vi "Input_Sensors_Conveyor.vi"(10 "IR Upper Limit Threshold":dbl=3.0, 11 "IR Distance Threshold":dbl=5.0) -> (0 "Conveyor Sensor Inputs":T2, 3 "ConveyorV2 Inputs":T1)   [LabVIEW 2012]
uses:
  Sensor_Input_Conveyor.ctl
  Sensor_Input_ConveyorV2.ctl
panel:
  out "error out":errorcluster
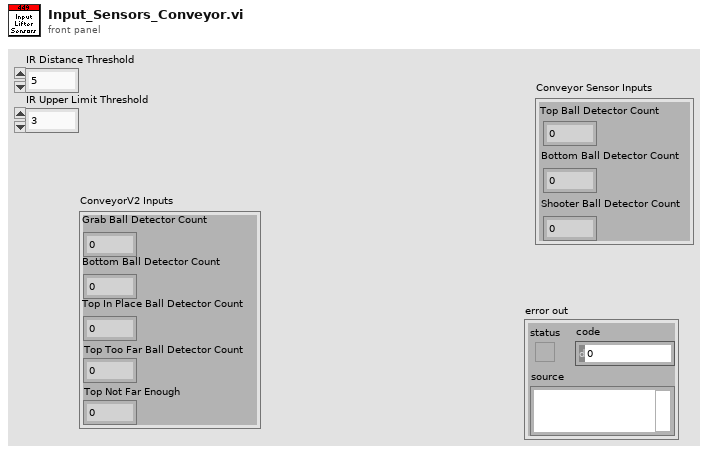
[diagram p1: front panel]
types:
  T1 = typedef "Sensor_Input_ConveyorV2.ctl" = cluster{"Grab Ball Detector Count":i32, "Bottom Ball Detector Count":i32, "Top In Place Ball Detector Count":i32, "Top Too Far Ball Detector Count":i32, "Top Not Far Enough":i32}
  T2 = typedef "Sensor_Input_Conveyor.ctl" = cluster{"Top Ball Detector Count":i32, "Bottom Ball Detector Count":i32, "Shooter Ball Detector Count":i32}
  T3 = typedef "WPI_DigitalInputDevRef.ctl" = cluster{"DevStatus":errorcluster, "DIO Channel":T4, "Digital Module":T5}
  T4 = typedef "FPGA_DIOChannel.ctl" = enum8{"DIO 1", "DIO 2", "DIO 3", "DIO 4", "DIO 5", "DIO 6", "DIO 7", "DIO 8", "DIO 9", "DIO 10", "DIO 11", "DIO 12", "DIO 13", "DIO 14", "Invalid"}
  T5 = typedef "FPGA_TypedefDigitalModule.ctl" = enum16{"Digital Module 1", "Digital Module 2"}
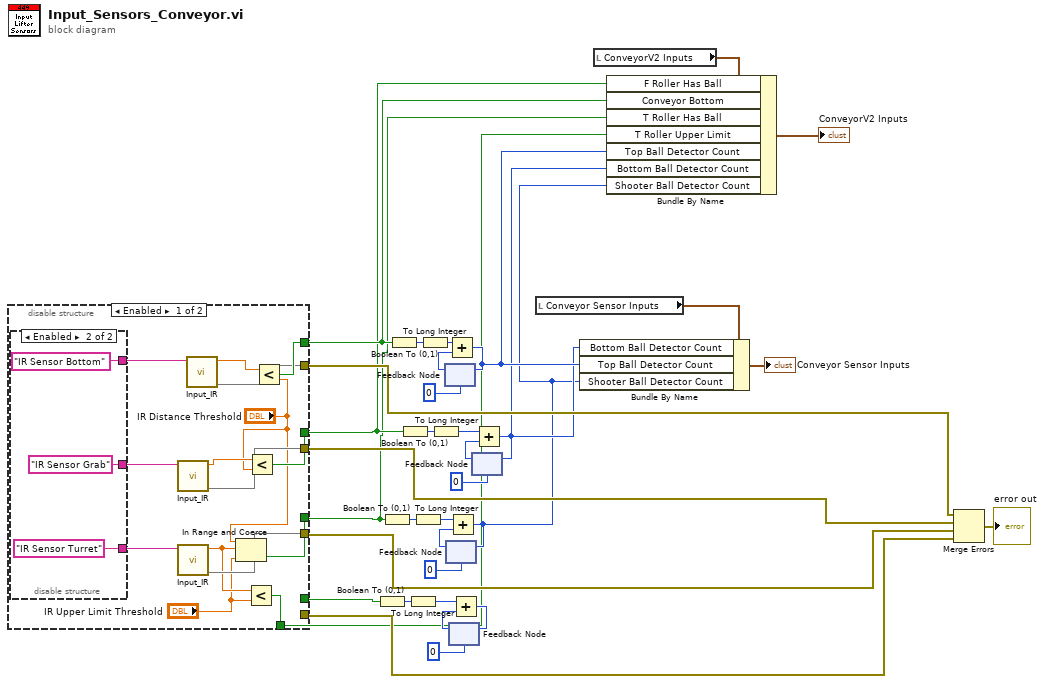
[diagram p0: block diagram]
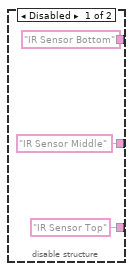
[diagram p2: hidden frame]
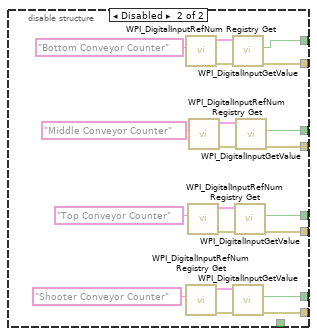
[diagram p3: hidden frame]
diagram:
  n1 = disable-structure shown="Enabled" {
    disable-tunnel: [w47 w72] -> w7
    disable-tunnel: [w44 w62] -> w4
    disable-tunnel: [w42 w61] -> w3
    disable-tunnel: [_ w60] -> w20
    disable-tunnel: [w45 w59] -> w19
    disable-tunnel: [w46 w58] -> w15
    disable-tunnel: [w41 w57] -> w18
    disable-tunnel: [_ w56] -> w17
    disable-tunnel: [w35 _] -> w1
    frame Enabled {
      n2 = disable-structure shown="Enabled" {
        disable-tunnel: ["IR Sensor Bottom" ("refnum name") "IR Sensor Bottom" ("Reference Name")] -> w49
        disable-tunnel: ["IR Sensor Top" ("refnum name") "IR Sensor Turret" ("Reference Name")] -> w43
        disable-tunnel: ["IR Sensor Middle" ("refnum name") "IR Sensor Grab" ("Reference Name")] -> w40
        frame Disabled {
        }
        frame Enabled {
        }
      }
      n3 = call "Input_IR.vi"("Analog Input"=w40) -> (0:w46, "Distance (in)"=w39:dbl)  [unwired: 9 in]
      n4 = call "Input_IR.vi"("Analog Input"=w43) -> (0:w41, "Distance (in)"=w37:dbl)  [unwired: 9 in]
      n5 = call "Input_IR.vi"("Analog Input"=w49) -> (0:w45, "Distance (in)"=w48:dbl)  [unwired: 9 in]
      n6 = In Range and Coerce(upper limit="IR Distance Threshold", x=w37, lower limit="IR Upper Limit Threshold") -> (In Range?=w42:bool)  [unwired: 1 out]
      n7 = Less?(x=w37, y="IR Upper Limit Threshold") -> (x < y?=w35:bool)
      n8 = Less?(x=w39, y="IR Distance Threshold") -> (x < y?=w44:bool)
      n9 = Less?(x=w48, y="IR Distance Threshold") -> (x < y?=w47:bool)
    }
    frame Disabled {
      n10 = call <vilib>:"WPI_DigitalInputRefNum Registry Get.vi"("refnum name"="Bottom Conveyor Counter") -> ("error out"=w73:errorcluster, "DigitalInputDevRef"=w74:T3)  [unwired: 9 in]
      n11 = call <vilib>:"WPI_DigitalInputRefNum Registry Get.vi"("refnum name"="Shooter Conveyor Counter") -> ("error out"=w65:errorcluster, "DigitalInputDevRef"=w64:T3)  [unwired: 9 in]
      n12 = call <vilib>:"WPI_DigitalInputRefNum Registry Get.vi"("refnum name"="Top Conveyor Counter") -> ("error out"=w66:errorcluster, "DigitalInputDevRef"=w67:T3)  [unwired: 9 in]
      n13 = call <vilib>:"WPI_DigitalInputRefNum Registry Get.vi"("refnum name"="Middle Conveyor Counter") -> ("error out"=w71:errorcluster, "DigitalInputDevRef"=w70:T3)  [unwired: 9 in]
      n14 = call <vilib>:"WPI_DigitalInputGetValue.vi"("error in (no error)"=w73, "DigitalInputDevRef"=w74) -> ("error out"=w59:errorcluster, "Value"=w72:bool)  [unwired: 7 in, 1 out]
      n15 = call <vilib>:"WPI_DigitalInputGetValue.vi"("error in (no error)"=w65, "DigitalInputDevRef"=w64) -> ("error out"=w56:errorcluster, "Value"=w60:bool)  [unwired: 7 in, 1 out]
      n16 = call <vilib>:"WPI_DigitalInputGetValue.vi"("error in (no error)"=w66, "DigitalInputDevRef"=w67) -> ("error out"=w57:errorcluster, "Value"=w61:bool)  [unwired: 7 in, 1 out]
      n17 = call <vilib>:"WPI_DigitalInputGetValue.vi"("error in (no error)"=w71, "DigitalInputDevRef"=w70) -> ("error out"=w58:errorcluster, "Value"=w62:bool)  [unwired: 7 in, 1 out]
    }
  }
  n18 = Boolean To (0,1)(Boolean=w20) -> (0, 1=w21:i16)
  n19 = Boolean To (0,1)(Boolean=w3) -> (0, 1=w28:i16)
  n20 = Boolean To (0,1)(Boolean=w7) -> (0, 1=w32:i16)
  n21 = Boolean To (0,1)(Boolean=w4) -> (0, 1=w11:i16)
  n22 = To Long Integer(number=w21) -> (32bit integer=w24:i32)
  n23 = To Long Integer(number=w28) -> (32bit integer=w25:i32)
  n24 = To Long Integer(number=w32) -> (32bit integer=w29:i32)
  n25 = To Long Integer(number=w11) -> (32bit integer=w14:i32)
  n26 = feedback #1(0) -> (w31:i32)
  n27 = feedback #2(0) -> (w27:i32)
  n28 = Add(x=w29, y=w31) -> (x+y=w6:i32)
  n29 = feedback-in #1(w6) -> ()
  n30 = Add(x=w25, y=w27) -> (x+y=w2:i32)
  n31 = feedback-in #2(w2) -> ()
  n32 = feedback #3(0) -> (w22:i32)
  n33 = Add(x=w24, y=w22) -> (x+y=w8:i32)
  n34 = feedback-in #3(w8) -> ()
  n35 = feedback #4(0) -> (w12:i32)
  n36 = Add(x=w14, y=w12) -> (x+y=w5:i32)
  n37 = feedback-in #4(w5) -> ()
  n38 = local read "Conveyor Sensor Inputs"() -> (w33:T2)
  n39 = Bundle By Name(cluster=w33, "Bottom Ball Detector Count"=w5, "Top Ball Detector Count"=w6, "Shooter Ball Detector Count"=w2) -> (→"Conveyor Sensor Inputs":T2)
  n40 = local read "ConveyorV2 Inputs"() -> (w9:T1)
  n41 = Bundle By Name(cluster=w9, "F Roller Has Ball"=w4, "Conveyor Bottom"=w7, "T Roller Has Ball"=w3, "T Roller Upper Limit"=w1, "Top Ball Detector Count"=w6, "Bottom Ball Detector Count"=w5, "Shooter Ball Detector Count"=w2) -> (→"ConveyorV2 Inputs":T1)
  n42 = Merge Errors(w19, w15, w18, w17) -> (→"error out":errorcluster)
